vi "SVM_Train_FromFile.vi"() -> (0 "error out":errorcluster, 3 "Model":T2)   [LabVIEW 2014]
uses:
  Controls/Kernel.ctl
  Wrapper API/Controls/svm_kernel_type.ctl
  Controls/Options Training.ctl
  Controls/Parameters NU_SVC.ctl
  Wrapper API/Controls/svm_model.ctl
  Wrapper API/Controls/svm_parameter.ctl
  Wrapper API/Controls/svm_type.ctl
  Wrapper API/Controls/svm_node.ctl
  Tools/Controls/Binary_ConfusionMatrix.ctl
  Logger/Controls/GFV Action.ctl
  SubVIs/SVM Train NU_SVC.vi
  Tools/SubVIs/Sparse - Scale Nodes Linear.vi
  <userlib>/_OpenG.lib/error/error.llb/Filter Error Codes (Array)__ogtk.vi
  Tools/SubVIs/Sparse - Scale Problem Linear.vi
  Wrapper API/svm_train.vi
  Wrapper API/svm_predict.vi
panel:
  out "Binary Confusion Matrix":T1
  in  "nu":T7=0.2 caption="nu (0,5)"
  in  "Options":T8={"cache_size"=500.0, "eps"=0.001, "shrinking"=TRUE, "probability"=FALSE}
  in  "Kernel":T9
  out "Logging output":string
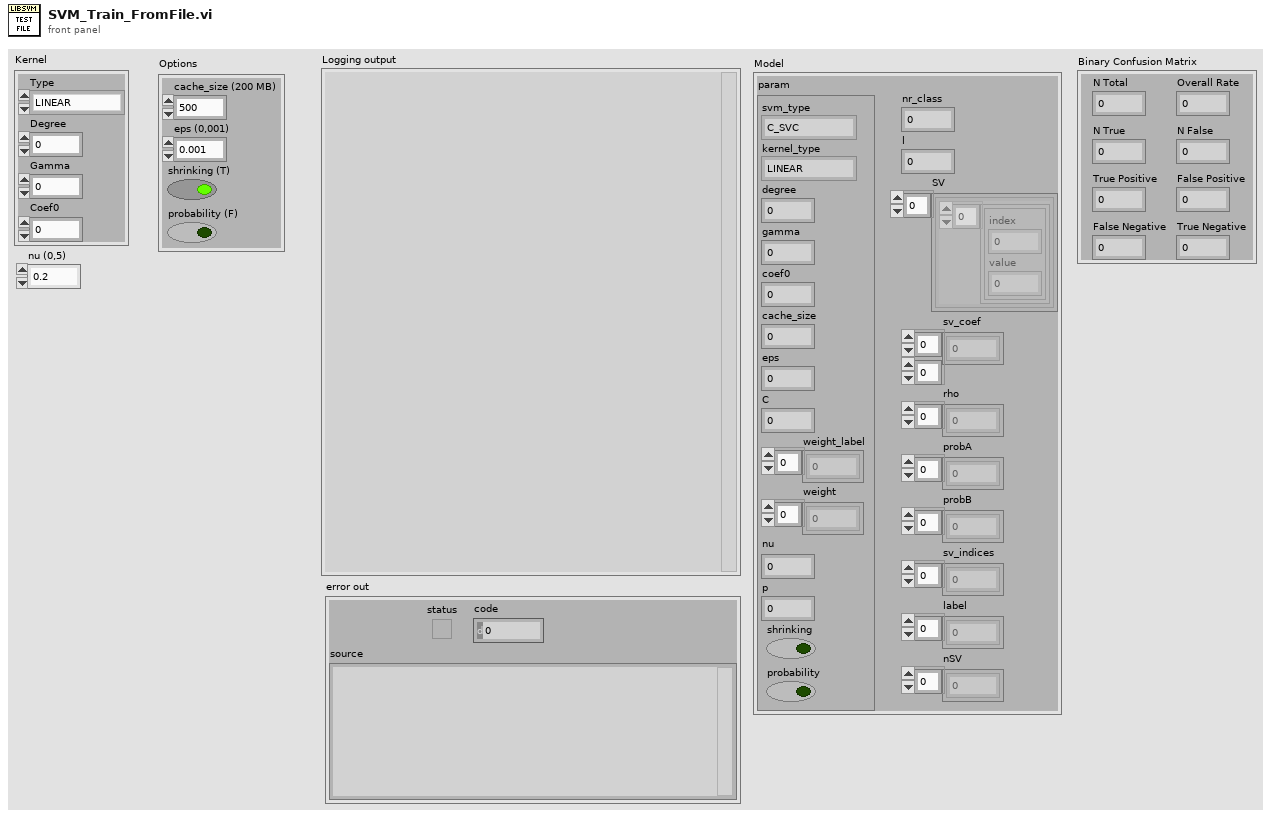
[diagram p1: front panel]
types:
  T1 = typedef "Binary_ConfusionMatrix.ctl" = cluster{"N Total":u32, "N True":u32, "N False":u32, "Overall Rate":dbl, "True Positive":dbl, "False Positive":dbl, "False Negative":dbl, "True Negative":dbl}
  T2 = typedef "svm_model.ctl" = cluster{"param":T3, "nr_class":i32, "l":i32, "SV":cluster{"Array":T6[]}[], "sv_coef":dbl[][], "rho":dbl[], "probA":dbl[], "probB":dbl[], "sv_indices":i32[], "label":i32[], "nSV":i32[]}
  T3 = typedef "svm_parameter.ctl" = cluster{"svm_type":T4, "kernel_type":T5, "degree":i32, "gamma":dbl, "coef0":dbl, "cache_size":dbl, "eps":dbl, "C":dbl, "weight_label":i32[], "weight":dbl[], "nu":dbl, "p":dbl, "shrinking":bool, "probability":bool}
  T4 = typedef "svm_type.ctl" = enum32{"C_SVC", "NU_SVC", "ONE_CLASS", "EPSILON_SVR", "NU_SVR"}
  T5 = typedef "svm_kernel_type.ctl" = enum32{"LINEAR", "POLY", "RBF", "SIGMOID", "PRECOMPUTED"}
  T6 = typedef "svm_node.ctl" = cluster{"index":i32, "value":dbl}
  T7 = typedef "Parameters NU_SVC.ctl" = dbl
  T8 = typedef "Options Training.ctl" = cluster{"cache_size":dbl, "eps":dbl, "shrinking":bool, "probability":bool}
  T9 = typedef "Kernel.ctl" = cluster{"Type":T5, "Degree":i32, "Gamma":dbl, "Coef0":dbl}
  T10 = typedef "GFV Action.ctl" = enum16{"Get", "Set", "Delete"}
  T11 = typedef "Logging_MessageQueue.ctl" = cluster{"Time":timestamp, "message":string}
  T12 = typedef "svm_problem.ctl" = cluster{"y":dbl[], "x":cluster{T6[]}[]}
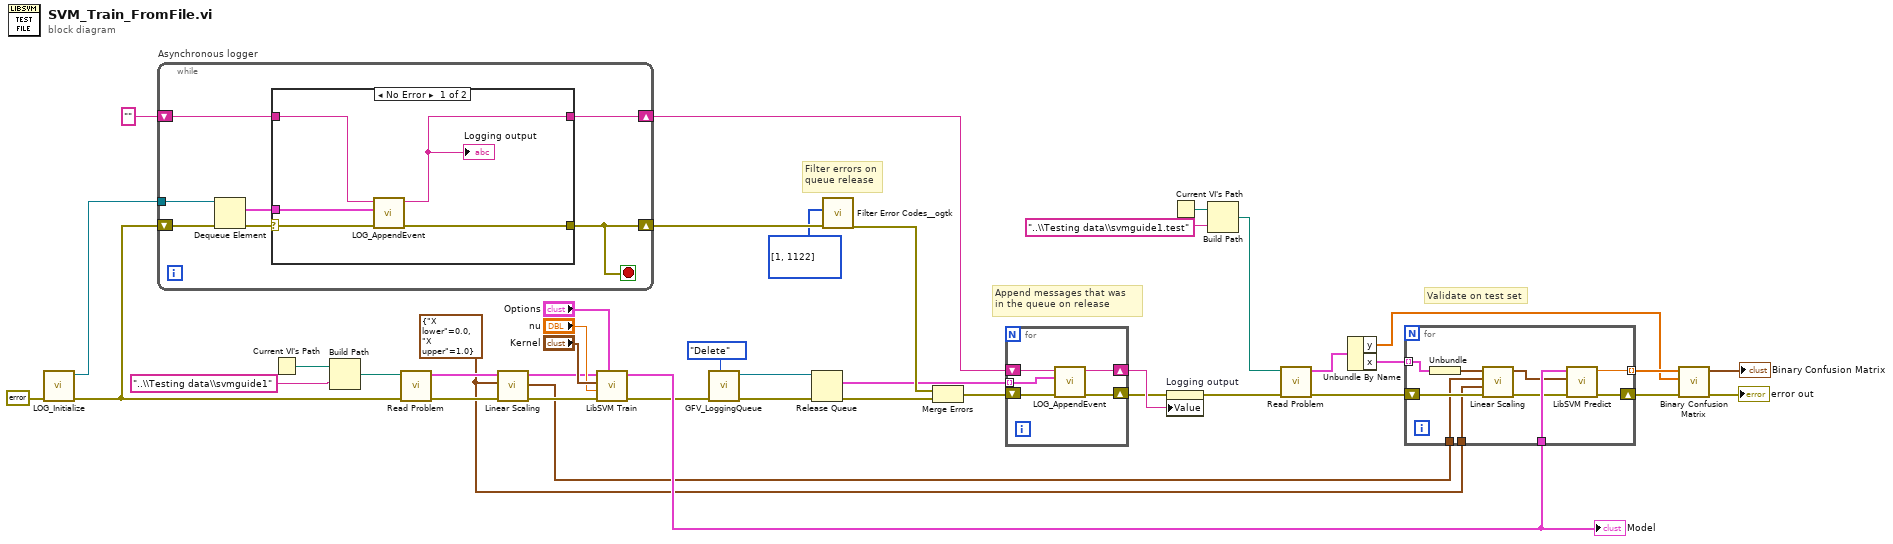
[diagram p0: block diagram]
diagram:
  w6 = cluster{"X lower":dbl, "X upper":dbl} {"X lower"=0.0, "X upper"=1.0} ("X Scaling limits")
  # "Validate on test set"
  # "Append messages that was \nin the queue on release"
  # "Filter errors on\nqueue release"
  n1 = call "LOG_Initialize.vi"("error in (no error)"=errorcluster {"status"=FALSE, "code"=0, "source"=""} ("error IO")) -> ("error out"=w37:errorcluster, "Message queue out"=w38:refnum<queue>)  [unwired: 9 in]
  n2 = while "Asynchronous logger" {
    tunnel: w38 -> [w49]
    shift-right: [w46] -> w30
    shift-left: "" -> [w45]
    shift-right: [w43] -> w35
    shift-left: w37 -> [w47]
    stop <- w43 stop-if-true
    n3 = Dequeue Element(queue=w49, error in (no error)=w47) -> (element=w48:T11, error out=w44:errorcluster)  [unwired: 1 in, 2 out]
    n4 = case shown="No Error" w44 {
      selector: w44 -> [w51 w56]
      tunnel: w48 -> [w54 _]
      tunnel: [w53 w55] -> w46
      tunnel: w45 -> [w52 w55]
      tunnel: [w50 w56] -> w43
      frame No Error {
        n5 = call "LOG_AppendEvent.vi"("error in (no error)"=w51, "Log Event"=w54, "String in"=w52) -> ("error out"=w50:errorcluster, "String out"=w53:string)  [unwired: 7 in]
        "Logging output" <- w53
      }
      frame Error {
      }
    }
  }
  n6 = Current VI's Path() -> (path=w20:path)
  n7 = Build Path(base path=w20, name or relative path="..\\Testing data\\svmguide1") -> (appended path=w40:path)
  n8 = call "Read Problem.vi"("error in (no error)"=w37, "file path (use dialog)"=w40) -> ("error out"=w10:errorcluster, "svm_problem"=w11:T12)  [unwired: 8 in]
  n9 = call-poly "Linear Scaling.vi"("error in (no error)"=w10, "X Scaling limits"=w6, "Problem"=w11) -> ("error out"=w9:errorcluster, "xmaxmin"=w7:cluster{"min":dbl, "max":dbl}[], "Scaled problem"=w8:T12)  [unwired: 5 in, 1 out]
  n10 = call-poly "LibSVM Train.vi"("Options"="Options", "error in (no error)"=w9, "nu"="nu", "Kernel"="Kernel", "Problem"=w8) -> ("error out"=w24:errorcluster, "Model"=w42:T2)  [unwired: 5 in]
  "Model" <- w42
  n11 = call "GFV_LoggingQueue.vi"("GFV Action"=GFV_Action."Delete", "error in (no error)"=w24) -> ("error out"=w27:errorcluster, "Message queue out"=w26:refnum<queue>)  [unwired: 8 in]
  n12 = Release Queue(queue=w26, error in (no error)=w27) -> (remaining elements=w32:T11[], error out=w36:errorcluster)  [unwired: 1 in, 1 out]
  n13 = call-poly <userlib>:"Filter Error Codes__ogtk.vi"("Error In"=w35, "Error Codes to Filter"=i32[] [1, 1122]) -> ("Error Out"=w34:errorcluster)  [unwired: 7 in, 2 out]
  n14 = Merge Errors(w34, w36) -> (w31:errorcluster)
  n15 = for {
    tunnel: w32 -> [w60] mode=indexing
    shift-right: [w58] -> w28
    shift-left: w31 -> [w61]
    shift-right: [w57] -> w29
    shift-left: w30 -> [w59]
    n16 = call "LOG_AppendEvent.vi"("error in (no error)"=w61, "Log Event"=w60, "String in"=w59) -> ("error out"=w58:errorcluster, "String out"=w57:string)  [unwired: 7 in]
  }
  n17 = property on="Logging output" class="Str"(error in=w28, "Value"=w29) -> (error out=w16:errorcluster)  [unwired: 1 in, 1 out]
  n18 = Current VI's Path() -> (path=w14:path)
  n19 = Build Path(base path=w14, name or relative path="..\\Testing data\\svmguide1.test") -> (appended path=w13:path)
  n20 = call "Read Problem.vi"("error in (no error)"=w16, "file path (use dialog)"=w13) -> ("error out"=w12:errorcluster, "svm_problem"=w18:T12)  [unwired: 8 in]
  n21 = Unbundle By Name(w18) -> ("y"=w3:dbl[], "x"=w17:cluster{T6[]}[])
  n22 = for {
    tunnel: w17 -> [w69] mode=indexing
    tunnel: [w71] -> w4 mode=indexing
    tunnel: w42 -> [w70]
    tunnel: w7 -> [w65]
    tunnel: w6 -> [w64]
    shift-right: [w63] -> w5
    shift-left: w12 -> [w68]
    n23 = Unbundle(w69) -> (w67:T6[])
    n24 = call-poly "Linear Scaling.vi"("error in (no error)"=w68, "Scaling limits"=w64, "xmaxmin"=w65, "x"=w67) -> ("error out"=w66:errorcluster, "x scaled"=w62:T6[])  [unwired: 6 in]
    n25 = call-poly "LibSVM Predict.vi"("error in (no error)"=w66, "X"=w62, "Model"=w70) -> ("error out"=w63:errorcluster, "Predicted label"=w71:dbl)  [unwired: 7 in]
  }
  n26 = call "Binary Confusion Matrix.vi"("error in (no error)"=w5, "Actual Labels"=w3, "Predicted Labels"=w4) -> ("error out"=→"error out":errorcluster, "Binary Confusion Matrix"=→"Binary Confusion Matrix":T1)  [unwired: 7 in]
